vi "Main v1.95.vi"() -> ()   [LabVIEW 2017]
doc: "v0.85:\n- Counts for rejects and total\n\nv0.5:\n\n- Added Reject to Manual Mode\n- Send reject pallet cluster during manual mode\n- Run continuous manual happens only when no error has occured"
uses:
  Controls/Main Tabs v0.1.ctl
  Controls/Auto.ctl
  RT/Controls/Auto Delays.ctl
  RT/Controls/Auto Times.ctl
  support/Controls/General Para.ctl
  Controls/UI Data.ctl
  Controls/AVL Auto Time.ctl
  support/Controls/Auto Stats.ctl
  Controls/Logging FGV.ctl
  support/Message Queue/Enqueue Message (Single).vi
  GV/Maintenance GV.vi
  <vilib>/Utility/error.llb/Error Cluster From Error Code.vi
  <vilib>/ErrorRing/Error Ring.xnode
  support/Message Queue/Message Queue.lvlib
  support/User Event - Stop/User Event - Stop.lvlib
panel:
  out "Rejects 2":u32 caption="Rejects"
  in  "Reset MCount":bool
  out "Output Count":u32 caption="Output\nCount"
  out "OEE":dbl format="%#.1f"
  out "QUA":dbl=100.0 min=0.0 max=100.0 step=0.1
  in  "Ideal Time":dbl=2.0 min=0.0 max=100.0 step=0.1
  in  "AVL":dbl=100.0 min=0.0 max=100.0 step=0.1
  out "PRF":dbl=100.0 min=0.0 max=100.0 step=0.1
  out "path":path
  out "Shutdown?":bool
  in  "Reject Pallets":T1
  out "Date-Time":string caption="Dip-Tube Assembly Automation (HMI) v1.95"
  out "Main Tab":T2
  in  "All IOs":bool
  in  "Autocycle":T3
  in  "Manual":bool
  in  "Parameters":bool
  in  "Maintenance":bool
  in  "General Para":T4={"Max. Cons."=5.0, "Offset 1"=0.0, "Offset 2"=0.0, "Offset 3"=0.0, "Offset 4"=0.0, "OutputPause"=0.0, "RejectPause"=0.0, "IndexTimeout"=0.0} caption="General" {"Offset 4" format="%.2f"; "Offset 3" format="%.2f"; "Offset 2" format="%.2f"; "Offset 1" format="%.2f"}
  in  "BF Para":cluster{"Delay 1":u32, "Delay 2":u32}={"Delay 1"=1000, "Delay 2"=1000}
  in  "Reject Para":cluster{"Delay":u32}={"Delay"=400}
  in  "PF Para":cluster{"Delay 1":u32, "Delay 2":u32}={"Delay 1"=1000, "Delay 2"=1000}
  in  "Tube Feeder Para":T5={"Delay"=400, "Delay 2"=250, "Max Attempts"=250, "Timeout"=8000} caption="TF Para"
  in  "Agitator Para":cluster{"Delay 1":u32, "Delay 2":u32}={"Delay 1"=400, "Delay 2"=250}
  in  "Insertion Para":cluster{"Delay 1":u32, "Delay 2":u32}={"Delay 1"=1000, "Delay 2"=1000}
  in  "Save Para":bool
  in  "Home Para":bool
  in  "Cutting Para":T6={"Delay"=400, "Delay 2"=250, "Delay 3"=250}
  in  "Meas. Para":T7={"Delay"=500.0, "Mean Length"=188.9, "Tolerance"=1.0}
  in  "Enable BF?":bool
  in  "Enable Agitate?":bool
  in  "Enable Reject?":bool
  in  "Toggle Motor":bool
  in  "Continuous?":bool
  in  "Enable Measure?":bool
  in  "Enable Index?":bool
  in  "Enable PF?":bool
  in  "Manual Para":T8={"Agitator Delays"=[400, 250], "TF Delays"=[700, 800, 2], "Insertion Delays"=[100, 500], "Cutting Delays"=[300, 300, 100], "PF Delays"=[250, 30000], "Measur. Delays"=[500.0, 188.9, 1.0], "Reject Delays"=[500], "BF Delays"=[1000, 1000]}
  in  "Enable Cutting?":bool
  in  "Enable Insertion?":bool
  in  "Run Manual":bool
  in  "Enable TF?":bool
  in  "Home Manual":bool
  out "Status 2":T10
  out "Measurements":T11 {"Height 1" format="%#.2f"; "Height 2" format="%#.2f"; "Height 3" format="%#.2f"; "Height 4" format="%#.2f"}
  in  "ResetRejectCount":bool
  in  "ResetGoodCount":bool
  out "RejectPause":u32 caption="Reject Parts"
  out "GoodPause":u32 caption="Good Parts"
  in  "End Cycle":bool
  out "Statuses":string[][](table)
  in  "All IO":bool
  in  "Stats":bool
  in  "Home AC":bool
  out "Status":string
  out "Good":u32 format="%06.0f"
  out "Cycle Time":dbl format="%0.2f"
  out "Rejects":u32 format="%05.0f"
  in  "View Log":bool
  out "Total Count 2":u32 caption="Total Count"
  out "Avg. Time":dbl caption="Avg. Cycle Time (s)" format="%#.3f"
  out "Output Chart":cluster{"Good Parts":u32, "Reject Parts":u32}(graph)
  out "Reject Count":u32
  out "Good Count":u32
  out "Total Time":dbl caption="Effective Cycle Time (s)" format="%#.3f"
  out "Time Chart":T12(graph)
  out "OEE Chart":T13(graph)
  out "Timestamp":string caption="Date & Timestamp"
  out "Latest Measure.":T14 caption="Latest Measurements" {"Length 1 (mm)" format="%#.2f"}
  out "Auto Times":T9
  in  "Back Stats":bool
  out "OEE 2":T13 caption="Latest Measurements" {"AVL" format="%#.1f"; "PRF" format="%#.1f"; "QUA" format="%#.1f"; "OEE" format="%#.1f"}
  out "Measurement Chart":T15(graph)
  in  "Home IOs":bool
  in  "Back IO":bool
  out "IAS 4":dbl format="%#.3f"
  out "IAS 3":dbl format="%#.3f"
  out "IAS 2":dbl format="%#.3f"
  out "IAS 1":dbl format="%#.3f"
  out "DI 1":T16
  out "DI 2":T17
  out "DO 1":T18
  in  "Exit":bool
  in  "Shutdown":bool
  # "HARMONY VISION DIP-TUBE ASSEMBLY AUTOMATION"
  # "Info"
  # "Delays: Time to wait (in milliseconds) after each action pertaining to each spcific station. Generally this timer starts after the required sensor that is expected either goes OFF or goes ON depending on the action. Some stations have multiple delays which are denoted by numbers relative to the sequence of action before the delay.\n\nTimeout: Maximum time allowed (in milliseconds) for a station to complete its actions.\n\nMax Attempts: Maximum number of attempts at retrying gate open/close.\n\nMean Length: Mean length of parts in the current model (in mm)\n\nTolerance: Acceptable deviation from mean length (in mm)\n\nMax Cons.: Maximum number of consecutive tubes missing on a particular pallet (as detected on measurement station) that will trigger an error and cycle stop.\n\nOffset: Offset factor (in mm) added to the measurement result of each probe.\n\nOutputPause & RejectPause: Countdown of number of parts before triggering an Auto-Pause."
  # "Auto-Pause after"
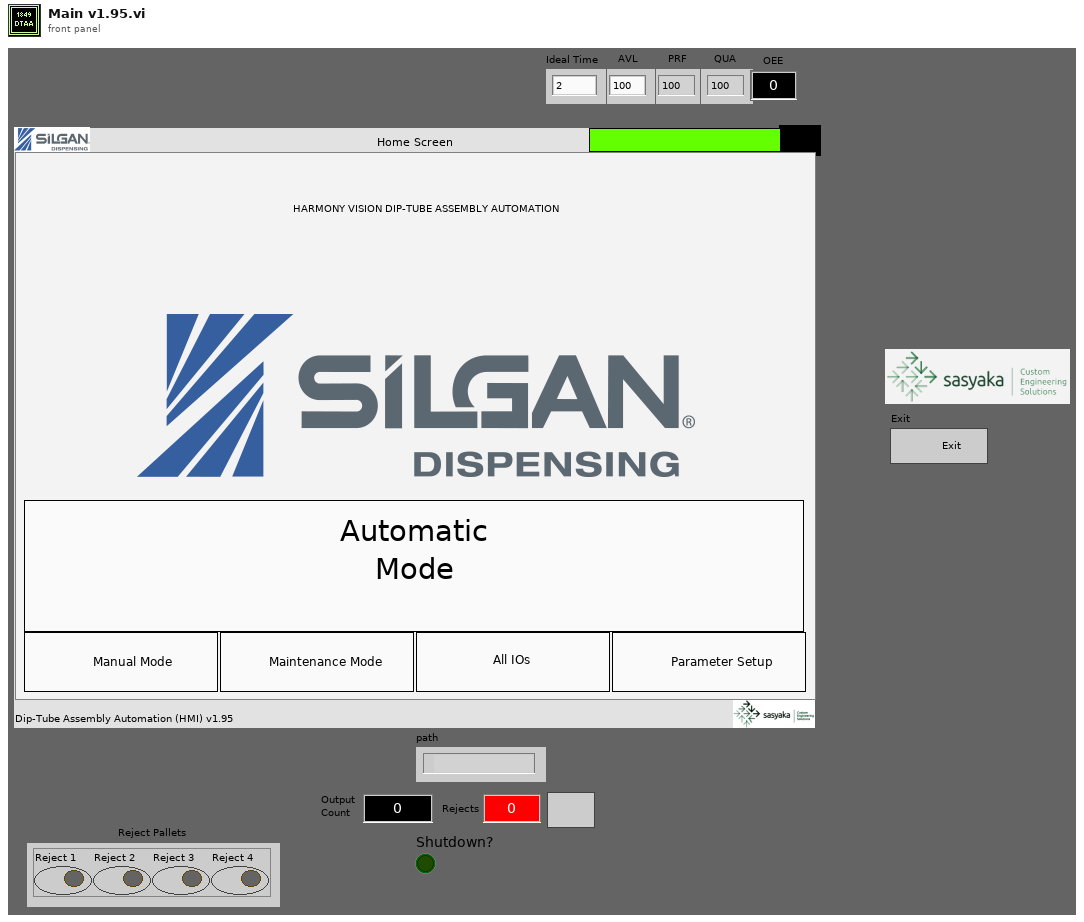
[diagram p1: front panel]
types:
  T1 = cluster{"Reject 1":bool, "Reject 2":bool, "Reject 3":bool, "Reject 4":bool}
  T2 = typedef "Main Tabs v0.1.ctl" = enum32{"Home Screen", "Parameter Setup", "Manual Mode", "Autocycle", "Autocycle Statistics", "Autocycle IOs"}
  T3 = typedef "Auto.ctl" = bool
  T4 = typedef "General Para.ctl" = cluster{"Max. Cons.":dbl, "Offset 1":dbl, "Offset 2":dbl, "Offset 3":dbl, "Offset 4":dbl, "OutputPause":dbl, "RejectPause":dbl, "IndexTimeout":dbl}
  T5 = cluster{"Delay":u32, "Delay 2":u32, "Max Attempts":u32, "Timeout":u32}
  T6 = cluster{"Delay":u32, "Delay 2":u32, "Delay 3":u32}
  T7 = cluster{"Delay":dbl, "Mean Length":dbl, "Tolerance":dbl}
  T8 = typedef "Auto Delays.ctl" = cluster{"Agitator Delays":u32[], "TF Delays":u32[], "Insertion Delays":u32[], "Cutting Delays":u32[], "PF Delays":u32[], "Measur. Delays":dbl[], "Reject Delays":u32[], "BF Delays":u32[]}
  T9 = typedef "Auto Times.ctl" = cluster{"Index Time":u32, "TF Time":u32, "Insertion Time":u32, "Cutting Time":u32, "PF Time":u32, "Meas. Time":u32, "Reject Time":u32}
  T10 = cluster{"Auto Times":T9, "error out":errorcluster}
  T11 = cluster{"Height 1":dbl, "Height 2":dbl, "Height 3":dbl, "Height 4":dbl}
  T12 = cluster{"Index":dbl, "TF":dbl, "Insert":dbl, "Cutting":dbl, "PF":dbl, "Measure.":dbl, "Reject":dbl, "Avg. Cycle Time":dbl}
  T13 = cluster{"AVL":dbl, "PRF":dbl, "QUA":dbl, "OEE":dbl}
  T14 = cluster{"Length 1 (mm)":dbl, "Pallet 2 (mm)":dbl, "Pallet 3 (mm)":dbl, "Pallet 4 (mm)":dbl}
  T15 = cluster{"1":dbl, "2":dbl, "3":dbl, "4":dbl, "4":dbl, "4":dbl}
  T16 = cluster{"Machine_ON":bool, "E_stop ":bool, "SW_Pressure":bool, "SW_Start ":bool, "SW_Reset":bool, "SW_Stop":bool, "SW_Door":bool, "RS_Index_Rotary_CW":bool, "RS_Index_Rotary_CCW":bool, "RS_Index_Stopper _Rear":bool, "RS_Index_Output_Separator_Rear":bool, "PES_Index_Pallet_Sensor":bool, "PES_Index_Output_Part Sensor":bool, "ICS_BF_Low_Level_1":bool, "ICS_BF_Low_Level_2":bool, "ICS_BF_Pump_CNVR_Full_1":bool, "ICS_BF_Pump_CNVR_Full_2":bool, "ICS_BF_Pump_CNVR_Full_3":bool, "ICS_BF_Pump_CNVR_Full_4":bool, "PES_PC_Pump Presence_1":bool, "PES_PC_Pump Presence_2":bool, "PES_PC_Pump Presence_3":bool, "PES_PC_Pump Presence_4":bool, "RS_PC_Gating_Front":bool, "PES_Pump_Interference":bool, "PES_TF_Low_Level":bool, "PES_Tube Presence_1":bool, "PES_Tube Presence_2":bool, "PES_Tube Presence_3":bool, "PES_Tube Presence_4":bool, "DI1.30":bool, "DI1.31":bool}
  T17 = cluster{"RS_Agitatator_1_Rear ":bool, "RS_Agitatator_2_Rear ":bool, "RS_TF_Gating CYL_Rear":bool, "RS_Insertion_1_Rear":bool, "RS_Insertion_1_Front":bool, "RS_Insertion _2_Rear":bool, "RS_Insertion _2_Front":bool, "RS_Insertion _3_Rear":bool, "RS_Insertion _3_Front":bool, "RS_Insertion _4_Rear":bool, "RS_Insertion _4_Front":bool, "RS_Insertion_Clamp_Rear":bool, "RS_Cutting_Rear":bool, "RS_Cutting_Clamp _Rear":bool, "RS_Measurement_1_Rear":bool, "RS_Measurement_2_Rear":bool, "RS_Measurement_3_Rear":bool, "RS_Measurement_4_Rear":bool, "DI2.18":bool, "RS_Rejection_1_Rear":bool, "RS_Rejection_2_Rear":bool, "RS_Rejection_3_Rear":bool, "RS_Rejection_4_Rear":bool, "DI2.23":bool, "DI2.24":bool, "DI2.25":bool, "DI2.26":bool, "DI2.27":bool, "DI2.28":bool, "DI2.29":bool, "DI2.30":bool, "DI2.31":bool}
  T18 = cluster{"TL_Red":bool, "TL_Orange":bool, "TL_Green":bool, "TL_Buzzer":bool, "SOL_Index_Rotary_CW":bool, "SOL_Index_Rotary_CCW":bool, "SOL_Index_Stopper_Rear":bool, "SOL_OutputSeparator_Rear":bool, "Bowl  Feeder_ ON 1":bool, "Pump_CNVR_Motor _ON":bool, "SOL_PC_Gating_CYL_Rear":bool, "SOL_Tube_Feed_Agitatator":bool, "SOL_Tube_Feed_Gating_CYL":bool, "SOL_Insertion _CYL":bool, "SOL_Insertion_Clamp_CYL":bool, "SOL_Cutting_CYL":bool, "SOL_Cutting_Clamp_CYL":bool, "SOL_Insertion_Air_Nozzle":bool, "SOL_Measurement_CYL":bool, "DO1.19":bool, "SOL_Rejection CYL_1":bool, "SOL_Rejection CYL_2":bool, "SOL_Rejection CYL_3":bool, "SOL_Rejection CYL_4":bool, "Bowl  Feeder_ ON 2":bool, "SOL_BF_BlowerON":bool, "SOL_BF1_Track1":bool, "SOL_BF1_Track2":bool, "SOL_BF2_Track1":bool, "SOL_BF2_Track2":bool, "DO1.30":bool, "DO1.31":bool}
  T19 = typedef "UI Data.ctl" = cluster{"Main Tab":refnum<vi>}
  T20 = typedef "Message Queue.lvlib/All Message Queues.ctl" = cluster{"UI":refnum<queue>}
  T21 = enum8{"Enabled", "Disabled", "Disabled and Grayed Out"}
  T22 = typedef "AVL Auto Time.ctl" = enum16{"Start Session", "Exited Auto", "Resumed Auto", "Read Time", "Reload Values"}
  T23 = cluster{"Array":string[][], "Machine Status":string}
  T24 = typedef "Logging FGV.ctl" = enum16{"Start Shift", "Reload Values", "Log Index", "Read Shift", "Close Shift", "Save Values"}
  T25 = typedef "Auto Stats.ctl" = cluster{"Time-Stamp":timestamp, "Auto Times":T9, "Measurements":cluster{"1":dbl, "2":dbl, "3":dbl, "4":dbl}, "Outputs":cluster{"Good Parts":u32, "Reject Parts":u32}, "Cycle Time":dbl, "Remarks":string}
  T26 = cluster{"Auto Times":T9, "Results":cluster{"Measurements":cluster{"1":dbl, "2":dbl, "3":dbl, "4":dbl}, "Reject Pallets":cluster{"Reject 1":bool, "Reject 2":bool, "Reject 3":bool, "Reject 4":bool}}, "OutputCount":u32, "error out":errorcluster}
  T27 = enum8{"Information", "Error", "Successful", "Tips"}
  T28 = cluster{"Agitator Delays[0]":u32, "Agitator Delays[1]":u32}
  T29 = cluster{"TF Delays[0]":u32, "TF Delays[1]":u32, "TF Delays[2]":u32, "TF Delays[3]":u32}
  T30 = cluster{"Insertion Delays[0]":u32, "Insertion Delays[1]":u32}
  T31 = cluster{"Cutting Delays[0]":u32, "Cutting Delays[1]":u32, "Cutting Delays[2]":u32}
  T32 = cluster{"Measur. Delays[0]":dbl, "Measur. Delays[1]":dbl, "Measur. Delays[2]":dbl}
  T33 = typedef "All Inputs.ctl" = cluster{"DI 1":cluster{"Machine_ON":bool, "E_stop ":bool, "SW_Pressure":bool, "SW_Start ":bool, "SW_Reset":bool, "SW_Stop":bool, "SW_Door":bool, "RS_Index_Rotary_CW":bool, "RS_Index_Rotary_CCW":bool, "RS_Index_Stopper _Rear":bool, "RS_Cutting_DNClamp _Rear":bool, "PES_Index_Pallet_Sensor":bool, "PES_Index_Output_Part Sensor":bool, "ICS_BF_Low_Level_1":bool, "ICS_BF_Low_Level_2":bool, "ICS_BF_Pump_CNVR_Full_1":bool, "ICS_BF_Pump_CNVR_Full_2":bool, "ICS_BF_Pump_CNVR_Full_3":bool, "ICS_BF_Pump_CNVR_Full_4":bool, "PES_PC_Pump Presence_1":bool, "PES_PC_Pump Presence_2":bool, "PES_PC_Pump Presence_3":bool, "PES_PC_Pump Presence_4":bool, "RS_PC_Gating_Front":bool, "PES_Pump_Interference":bool, "PES_TF_Low_Level":bool, "PES_Tube Presence_1":bool, "PES_Tube Presence_2":bool, "PES_Tube Presence_3":bool, "PES_Tube Presence_4":bool, "DI1.30":bool, "DI1.31":bool}, "DI 2":cluster{"RS_Agitatator_1_Rear ":bool, "RS_Agitatator_2_Rear ":bool, "RS_TF_Gating CYL_Rear":bool, "RS_Insertion_1_Rear":bool, "RS_Insertion_1_Front":bool, "RS_Insertion _2_Rear":bool, "RS_Insertion _2_Front":bool, "RS_Insertion _3_Rear":bool, "RS_Insertion _3_Front":bool, "RS_Insertion _4_Rear":bool, "RS_Insertion _4_Front":bool, "RS_Insertion_Clamp_Rear":bool, "RS_Cutting_Rear":bool, "RS_Cutting_UPClamp _Rear":bool, "RS_Measurement_1_Rear":bool, "RS_Measurement_2_Rear":bool, "RS_Measurement_3_Rear":bool, "RS_Measurement_4_Rear":bool, "RS_Measure_Clamp_Rear":bool, "RS_Rejection_1_Rear":bool, "RS_Rejection_2_Rear":bool, "RS_Rejection_3_Rear":bool, "RS_Rejection_4_Rear":bool, "DI2.23":bool, "DI2.24":bool, "DI2.25":bool, "DI2.26":bool, "DI2.27":bool, "DI2.28":bool, "DI2.29":bool, "DI2.30":bool, "DI2.31":bool}, "IAS 1":dbl, "IAS 2":dbl, "IAS 3":dbl, "IAS 4":dbl, "DO 1":cluster{"TL_Red":bool, "TL_Orange":bool, "TL_Green":bool, "TL_Buzzer":bool, "SOL_Index_Rotary_CW":bool, "SOL_Index_CNVR_Rotary_CCW":bool, "SOL_Index_CNVR_Stopper_Rear":bool, "SOL_Index_CNVR_Output _Separator _Rear":bool, "Bowl  Feeder_ ON 1":bool, "Pump_CNVR_Motor _ON":bool, "SOL_PC_Gating_CYL_Rear":bool, "SOL_Tube_Feed_Agitatator":bool, "SOL_Tube_Feed_Gating_CYL":bool, "SOL_Insertion _CYL":bool, "SOL_Insertion_Clamp_CYL":bool, "SOL_Cutting_CYL":bool, "SOL_Cutting_Clamp_CYL":bool, "SOL_Insertion_Air_Nozzle":bool, "SOL_Measurement_CYL":bool, "DO1.19":bool, "SOL_Rejection CYL_1":bool, "SOL_Rejection CYL_2":bool, "SOL_Rejection CYL_3":bool, "SOL_Rejection CYL_4":bool, "Bowl  Feeder_ ON 2":bool, "SOL_BF_BlowerON":bool, "SOL_BF1_Track1":bool, "SOL_BF1_Track2":bool, "SOL_BF2_Track1":bool, "SOL_BF2_Track2":bool, "DO1.30":bool, "DO1.31":bool}}
  T34 = cluster{"Machine_ON":bool, "E_stop ":bool, "SW_Pressure":bool, "SW_Start ":bool, "SW_Reset":bool, "SW_Stop":bool, "SW_Door":bool, "RS_Index_Rotary_CW":bool, "RS_Index_Rotary_CCW":bool, "RS_Index_Stopper _Rear":bool, "RS_Cutting_DNClamp _Rear":bool, "PES_Index_Pallet_Sensor":bool, "PES_Index_Output_Part Sensor":bool, "ICS_BF_Low_Level_1":bool, "ICS_BF_Low_Level_2":bool, "ICS_BF_Pump_CNVR_Full_1":bool, "ICS_BF_Pump_CNVR_Full_2":bool, "ICS_BF_Pump_CNVR_Full_3":bool, "ICS_BF_Pump_CNVR_Full_4":bool, "PES_PC_Pump Presence_1":bool, "PES_PC_Pump Presence_2":bool, "PES_PC_Pump Presence_3":bool, "PES_PC_Pump Presence_4":bool, "RS_PC_Gating_Front":bool, "PES_Pump_Interference":bool, "PES_TF_Low_Level":bool, "PES_Tube Presence_1":bool, "PES_Tube Presence_2":bool, "PES_Tube Presence_3":bool, "PES_Tube Presence_4":bool, "DI1.30":bool, "DI1.31":bool}
  T35 = cluster{"RS_Agitatator_1_Rear ":bool, "RS_Agitatator_2_Rear ":bool, "RS_TF_Gating CYL_Rear":bool, "RS_Insertion_1_Rear":bool, "RS_Insertion_1_Front":bool, "RS_Insertion _2_Rear":bool, "RS_Insertion _2_Front":bool, "RS_Insertion _3_Rear":bool, "RS_Insertion _3_Front":bool, "RS_Insertion _4_Rear":bool, "RS_Insertion _4_Front":bool, "RS_Insertion_Clamp_Rear":bool, "RS_Cutting_Rear":bool, "RS_Cutting_UPClamp _Rear":bool, "RS_Measurement_1_Rear":bool, "RS_Measurement_2_Rear":bool, "RS_Measurement_3_Rear":bool, "RS_Measurement_4_Rear":bool, "RS_Measure_Clamp_Rear":bool, "RS_Rejection_1_Rear":bool, "RS_Rejection_2_Rear":bool, "RS_Rejection_3_Rear":bool, "RS_Rejection_4_Rear":bool, "DI2.23":bool, "DI2.24":bool, "DI2.25":bool, "DI2.26":bool, "DI2.27":bool, "DI2.28":bool, "DI2.29":bool, "DI2.30":bool, "DI2.31":bool}
  T36 = cluster{"TL_Red":bool, "TL_Orange":bool, "TL_Green":bool, "TL_Buzzer":bool, "SOL_Index_Rotary_CW":bool, "SOL_Index_CNVR_Rotary_CCW":bool, "SOL_Index_CNVR_Stopper_Rear":bool, "SOL_Index_CNVR_Output _Separator _Rear":bool, "Bowl  Feeder_ ON 1":bool, "Pump_CNVR_Motor _ON":bool, "SOL_PC_Gating_CYL_Rear":bool, "SOL_Tube_Feed_Agitatator":bool, "SOL_Tube_Feed_Gating_CYL":bool, "SOL_Insertion _CYL":bool, "SOL_Insertion_Clamp_CYL":bool, "SOL_Cutting_CYL":bool, "SOL_Cutting_Clamp_CYL":bool, "SOL_Insertion_Air_Nozzle":bool, "SOL_Measurement_CYL":bool, "DO1.19":bool, "SOL_Rejection CYL_1":bool, "SOL_Rejection CYL_2":bool, "SOL_Rejection CYL_3":bool, "SOL_Rejection CYL_4":bool, "Bowl  Feeder_ ON 2":bool, "SOL_BF_BlowerON":bool, "SOL_BF1_Track1":bool, "SOL_BF1_Track2":bool, "SOL_BF2_Track1":bool, "SOL_BF2_Track2":bool, "DO1.30":bool, "DO1.31":bool}
  T37 = cluster{"Index":dbl, "TF":dbl, "Insert":dbl, "Cutting":dbl, "PF":dbl, "Measure.":dbl, "Reject":dbl}
  T38 = cluster{"1":dbl, "2":dbl, "3":dbl, "4":dbl, dbl, dbl}
  T39 = cluster{"Manual Para":T8, "Reject Pallets":cluster{"Reject 1":bool, "Reject 2":bool, "Reject 3":bool, "Reject 4":bool}}
  T40 = cluster{"Measurements":cluster{"1":dbl, "2":dbl, "3":dbl, "4":dbl}, "Reject Pallets":cluster{"Reject 1":bool, "Reject 2":bool, "Reject 3":bool, "Reject 4":bool}}
  T41 = cluster{"Reject Pallets":cluster{"Reject 1":bool, "Reject 2":bool, "Reject 3":bool, "Reject 4":bool}, "Measurements":cluster{"1":dbl, "2":dbl, "3":dbl, "4":dbl}}
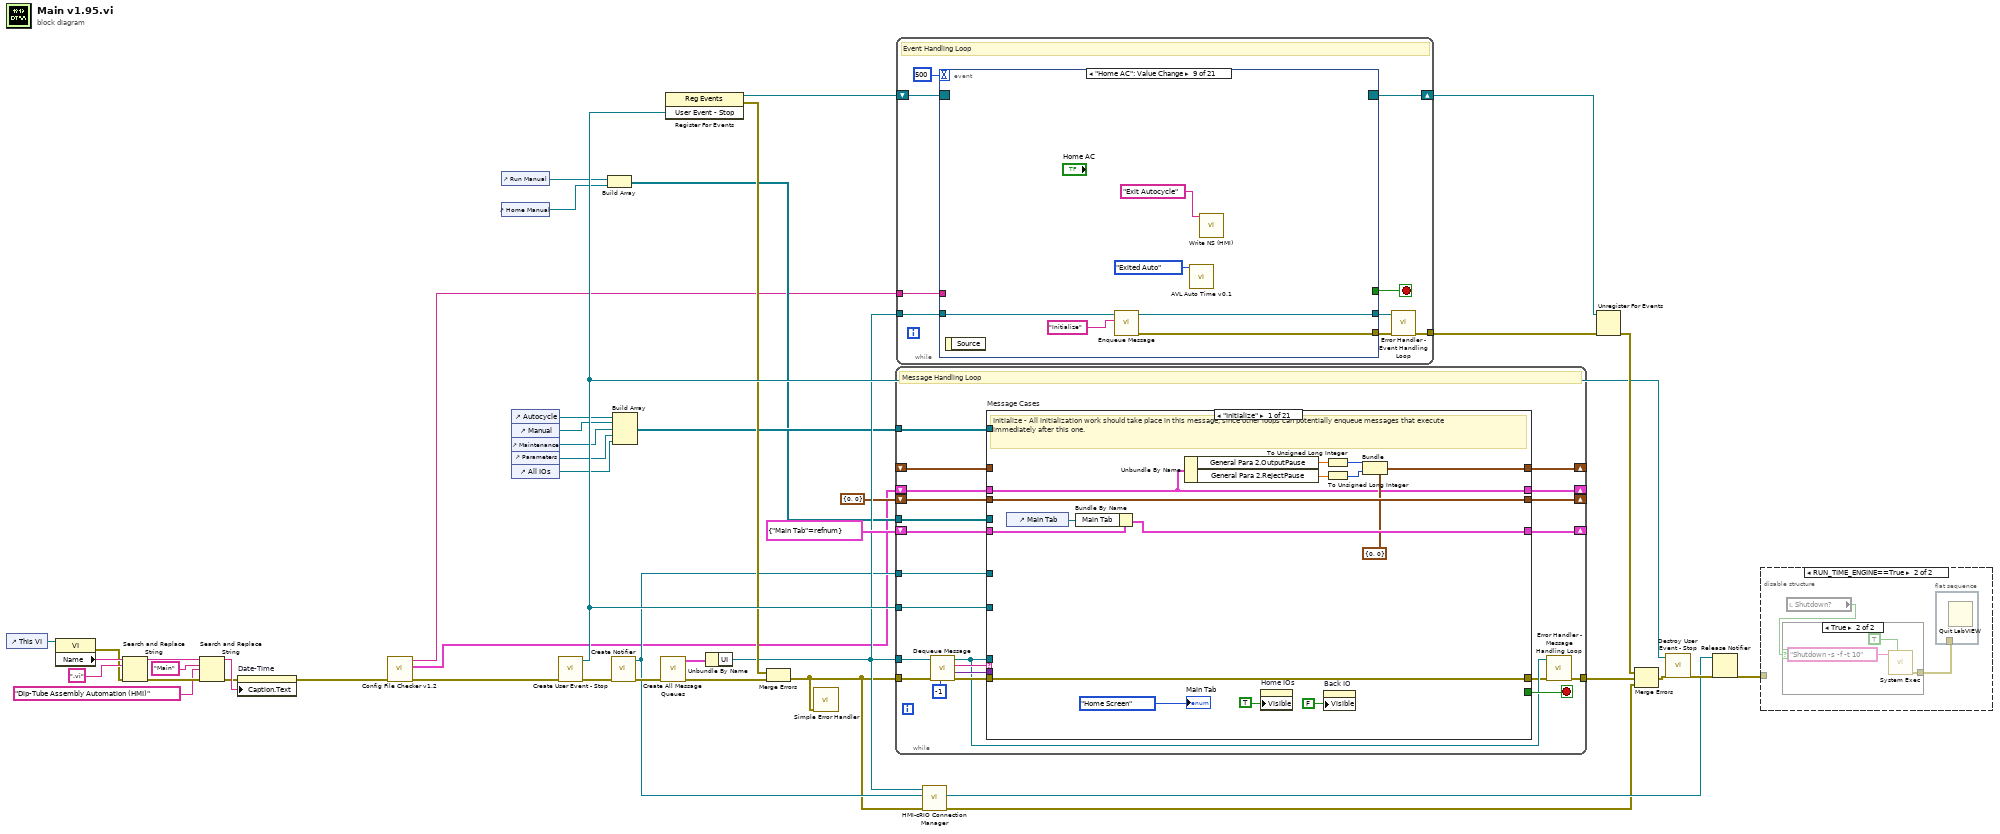
[diagram p0: block diagram]
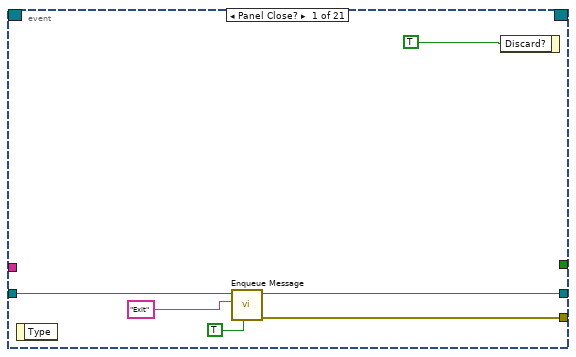
[diagram p2: hidden frame]
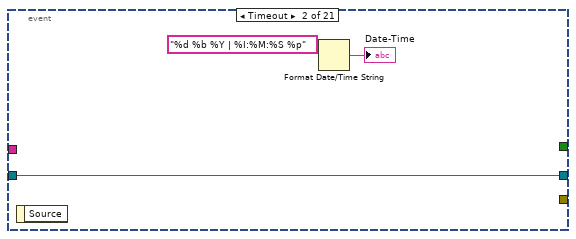
[diagram p3: hidden frame]
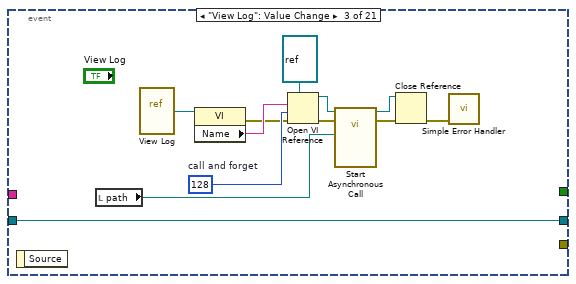
[diagram p4: hidden frame]
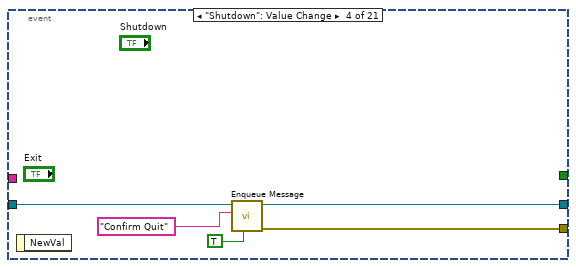
[diagram p5: hidden frame]
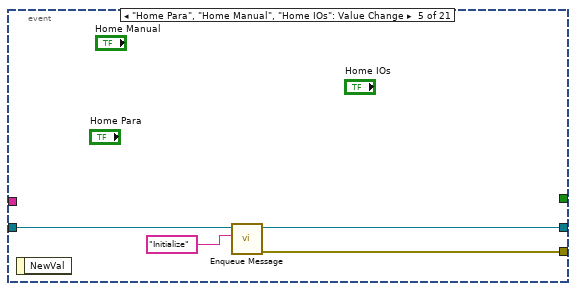
[diagram p6: hidden frame]
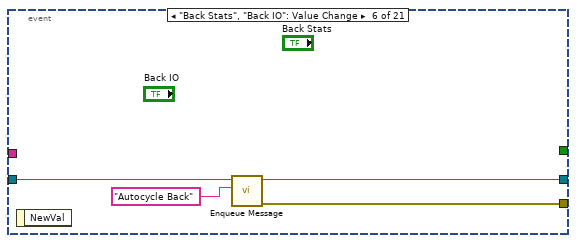
[diagram p7: hidden frame]
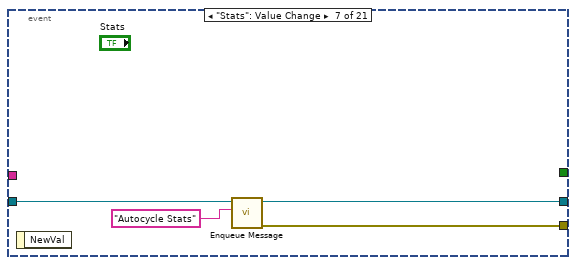
[diagram p8: hidden frame]
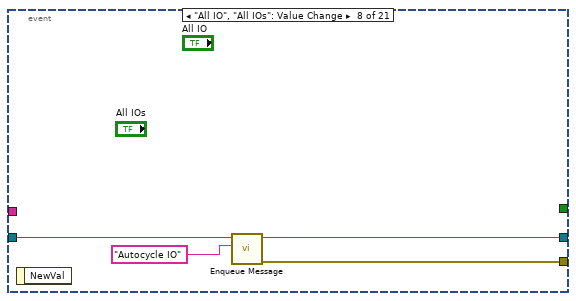
[diagram p9: hidden frame]
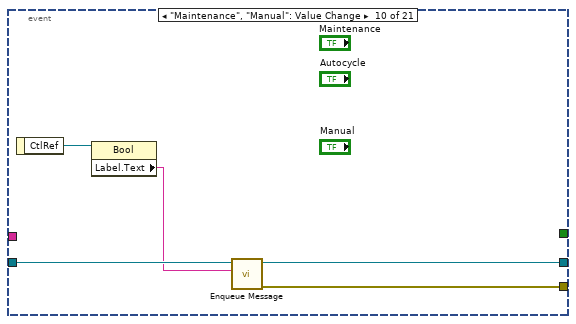
[diagram p10: hidden frame]
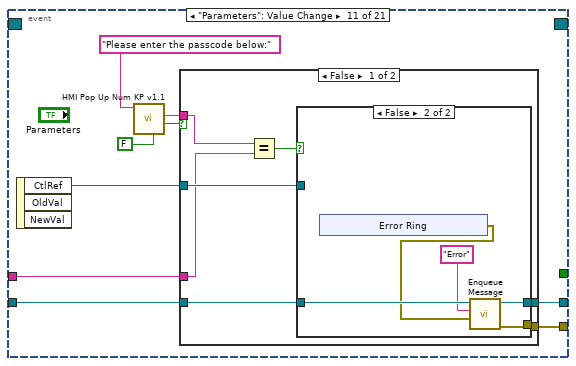
[diagram p11: hidden frame]
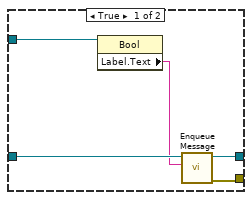
[diagram p12: hidden frame]
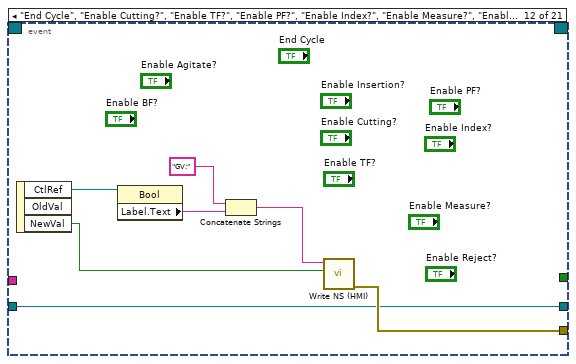
[diagram p14: hidden frame]
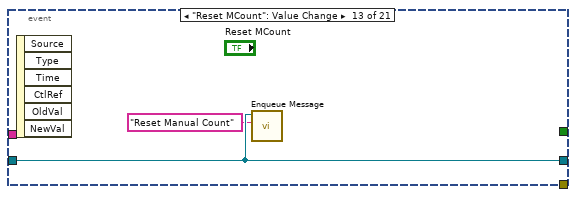
[diagram p15: hidden frame]
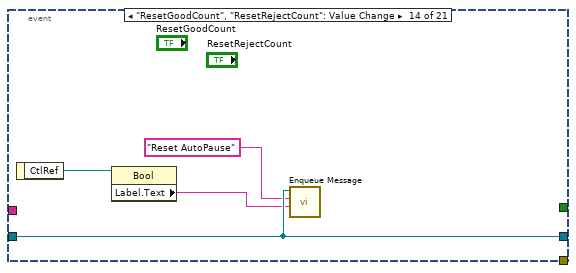
[diagram p16: hidden frame]
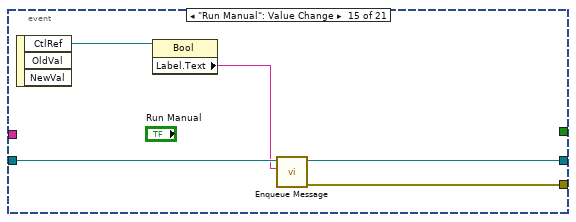
[diagram p17: hidden frame]
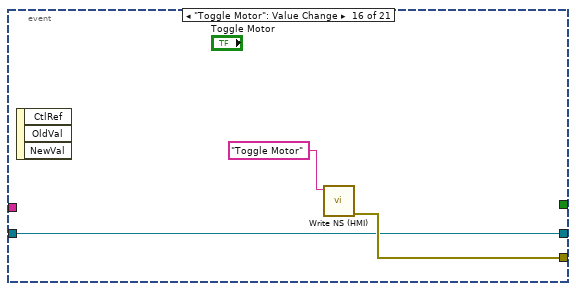
[diagram p18: hidden frame]
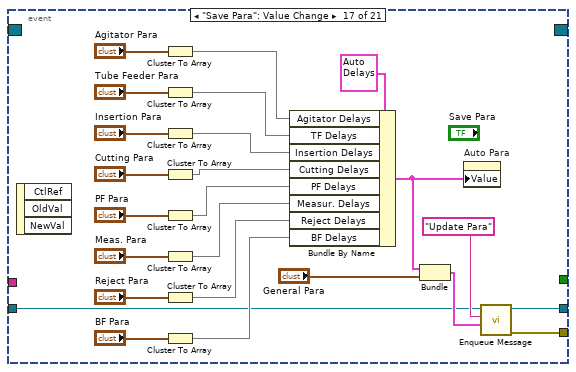
[diagram p19: hidden frame]
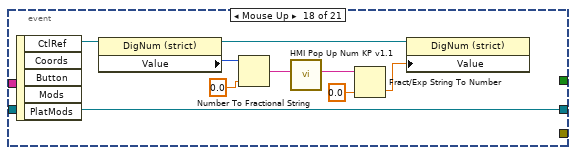
[diagram p20: hidden frame]
diagram:
  n1 = control-ref of="This VI"() -> (w15:refnum<vi>)
  n2 = property class="VI"(reference=w15) -> (error out=w14:errorcluster, "Name"=w21:string)  [unwired: 1 in, 1 out]
  n3 = Search and Replace String(input string=w21, search string=".vi", error in=w14) -> (result string=w19:string, error out=w18:errorcluster)  [unwired: 5 in, 2 out]
  n4 = Search and Replace String(input string=w19, search string="Main", replace string="Dip-Tube Assembly Automation (HMI)" ("replace string (\"\")"), error in=w18) -> (result string=w13:string, error out=w12:errorcluster)  [unwired: 4 in, 2 out]
  n5 = property on="Date-Time" class="Str"(error in=w12, "Caption.Text"=w13) -> (error out=w5:errorcluster)  [unwired: 1 in, 1 out]
  n6 = call "Config File Checker v1.2.vi"("Error In"=w5) -> ("error out"=w4:errorcluster, "All Para"=w1:cluster{"Auto Para":T8, "General Para 2":T4}, "password"=w3:string)  [unwired: 7 in, 1 out]
  n7 = control-ref of="Run Manual"() -> (w11:refnum<vi>)
  n8 = control-ref of="Home Manual"() -> (w10:refnum<vi>)
  n9 = control-ref of="Autocycle"() -> (w26:refnum<vi>)
  n10 = control-ref of="Manual"() -> (w25:refnum<vi>)
  n11 = control-ref of="Maintenance"() -> (w24:refnum<vi>)
  n12 = control-ref of="Parameters"() -> (w23:refnum<vi>)
  n13 = control-ref of="All IOs"() -> (w6:refnum<vi>)
  n14 = call "Create User Event - Stop.vi"("error in (no error)"=w4) -> ("error out"=w32:errorcluster, "User Event - Stop"=w35:refnum<user-event>)  [unwired: 9 in]
  n15 = Build Array(w11, w10) -> (w9:refnum<vi>[])
  n16 = call "Create Notifier.vi"("error in (no error)"=w32) -> ("error out"=w31:errorcluster, "notifier out"=w7:refnum<notifier>)  [unwired: 9 in]
  n17 = Build Array(w26, w25, w24, w23, w6) -> (w22:refnum<vi>[])
  n18 = call "Create All Message Queues.vi"("error in (no error)"=w31) -> ("error out"=w44:errorcluster, "Message Queues out"=w43:T20)  [unwired: 9 in]
  n19 = register-events(w35) -> (reference out=w36:refnum<event-registration>, error out=w34:errorcluster)  [unwired: 2 in]
  n20 = Unbundle By Name(w43) -> ("UI"=w33:refnum<queue>)
  n21 = Merge Errors(w34, w44) -> (w2:errorcluster)
  n22 = call <vilib>:"Simple Error Handler.vi"("error in (no error)"=w2) -> ()  [unwired: 4 in, 5 out]
  n23 = while {
    tunnel: w33 -> [w59]
    shift-right: [w66] -> _
    shift-left: T19 {"Main Tab"=refnum} ("Data Cluster") -> [w49]
    tunnel: w35 -> [w64]
    tunnel: w2 -> [w63]
    tunnel: [w57] -> w42
    tunnel: w7 -> [w54]
    tunnel: w22 -> [w53]
    tunnel: w9 -> [w52]
    shift-right: [w50] -> _
    shift-left: cluster{"OutputCount":u32, "RejectCount":u32} {"OutputCount"=0, "RejectCount"=0} -> [w51]
    shift-right: [w47] -> _
    shift-left: w1 -> [w48]
    shift-right: [w45] -> _
    shift-left: _ -> [w46]
    stop <- w65 stop-if-true
    # "Message Handling Loop"
    n24 = call "Dequeue Message.vi"("timeout"=-1, "error in (no error)"=w63, "Message Queue"=w59) -> ("error out"=w62:errorcluster, "Message Data"=w60:variant, "Message"=w61:string, "dup Message Queue"=w58:refnum<queue>)  [unwired: 5 in]
    n25 = case "Message Cases" shown="\"Initialize\"" w61 {
      selector: w61 -> [_ _ _ _ _ _ _ _ _ _ _ _ _ _ _ _ _ _ _ _ w470]
      tunnel: w58 -> [_ _ _ _ _ _ _ _ _ w225 w235 _ w280 _ w361 _ _ _ w438 w466 _]
      tunnel: w62 -> [w81 w86 w102 w132 w149 w167 w178 w211 w218 w227 w243 w273 w323 w335 w369 w381 w391 w428 w442 w459 _]
      tunnel: [w81 w85 w91 w132 w144 w167 w177 w211 w218 w226 w242 w274 w324 w337 w360 w381 w390 w423 w440 w462 w471] -> w56
      tunnel: w49 -> [w80 w87 w104 w136 w151 w166 w174 w215 w222 w232 w240 w275 w325 w338 w370 w380 w393 w427 w441 w465 w472]
      tunnel: [w79 w87 w104 w136 w151 w166 w174 w215 w222 w232 w240 w275 w325 w338 w370 w380 w393 w427 w441 w465 w472] -> w66
      tunnel: [_ _ _ _ _ _ _ _ _ _ _ _ _ _ _ _ _ _ _ TRUE _] -> w65
      tunnel: w60 -> [_ _ w101 _ w148 _ _ _ _ _ _ w272 w322 _ w368 _ w389 w426 _ w456 _]
      tunnel: w64 -> [_ _ _ _ _ _ _ _ _ _ _ _ _ _ _ _ _ _ _ w461 _]
      tunnel: w54 -> [_ _ _ _ _ _ _ _ _ _ _ _ _ _ _ _ _ _ _ w455 _]
      tunnel: w53 -> [_ _ w97 _ _ _ _ _ _ _ _ _ _ _ _ _ _ _ _ _ _]
      tunnel: w52 -> [_ _ _ _ _ _ _ _ _ _ _ _ _ w332 w366 _ _ _ _ _ _]
      tunnel: w51 -> [w76 w84 w93 w133 w150 w155 w179 w212 w219 w229 w244 w270 w320 w328 w359 _ w392 w422 w437 w452 w469]
      tunnel: [w76 w84 w93 w133 w150 w155 w179 w212 w219 w229 w244 w270 w320 w328 w354 cluster{"OutputCount":u32, "RejectCount":u32} {"OutputCount"=0, "RejectCount"=0} w392 w422 w437 w452 w469] -> w50
      tunnel: w48 -> [w68 w83 w90 w113 _ w154 w173 w210 w217 w224 w234 w259 w289 w327 w342 w377 w385 w405 w430 w451 w468]
      tunnel: [w68 w83 w90 w113 w143 w154 w173 w210 w217 w224 w234 w259 w289 w327 w342 w377 w385 w405 w430 w451 w468] -> w47
      tunnel: w46 -> [_ w82 w88 w112 w137 w152 w170 w209 w216 w223 w233 w258 w281 w326 w341 w376 w386 w404 w429 w450 w467]
      tunnel: [w67 w82 w88 w112 w137 w152 w171 w209 w216 w223 w233 w258 w278 w326 w341 w376 w384 w404 w429 w450 w467] -> w45
      frame "Initialize" {
        # "Initialize - All initialization work should take place in this message, since other loops can potentially enqueue messages that execute immediately after this one."
        n26 = control-ref of="Main Tab"() -> (w78:refnum<vi>)
        n27 = Bundle By Name(cluster=w80, "Main Tab"=w78) -> (w79:T19)
        n28 = Unbundle By Name(w68) -> ("General Para 2.OutputPause"=w71:dbl, "General Para 2.RejectPause"=w70:dbl)
        n29 = property on="Home IOs" class="Bool"("Visible"=TRUE) -> ()  [unwired: 2 in, 2 out]
        n30 = property on="Back IO" class="Bool"("Visible"=FALSE) -> ()  [unwired: 2 in, 2 out]
        n31 = To Unsigned Long Integer(number=w71) -> (unsigned 32bit integer=w72:u32)
        n32 = To Unsigned Long Integer(number=w70) -> (unsigned 32bit integer=w73:u32)
        n33 = Bundle(cluster=cluster{"GoodPause":u32, "RejectPause":u32} {"GoodPause"=0, "RejectPause"=0}, "GoodPause"=w72, "RejectPause"=w73) -> (w67:cluster{"GoodPause":u32, "RejectPause":u32})
        "Main Tab" <- Main_Tabs_v0.1."Home Screen" ("Main Tab")
      }
      frame "Maintenance" {
        # "Maintenance"
        n34 = call "Maintenance v0.3.vi"("Error In"=w86) -> ("Error out"=w85:errorcluster)  [unwired: 10 in]
      }
      frame "Connection" {
        n35 = Variant To Data(error in=w102, type=FALSE, Variant=w101) -> (data=w89:bool, error out=w92:errorcluster)
        n36 = Select(t=u32 6618880 ("Text.Text Colors:BG Color"), s=w89, f=u32 16762112 ("Text.Text Colors:BG Color")) -> (s? t:f=w98:u32)
        n37 = property on="Date-Time" class="Str"("Text.BGColor"=w98) -> ()  [unwired: 2 in, 2 out]
        n38 = Select(t=T21."Enabled" ("Disabled"), s=w89, f=T21."Disabled and Grayed Out") -> (s? t:f=w95:T21)
        n39 = for {
          tunnel: w97 -> [w111] mode=indexing
          tunnel: w95 -> [w110]
          n40 = property class="Bool"(reference=w111, "DisabledEnum"=w110) -> ()  [unwired: 1 in, 2 out]
        }
        n41 = case shown="True" w89 {
          tunnel: w92 -> [w105 w108]
          tunnel: [w105 w107] -> w91
          tunnel: w90 -> [_ w106]
          frame False {
          }
          frame True {
            n42 = call "Write NS (HMI).vi"("error in (no error)"=w108, "Message Data"=w106, "Message"="Save Para") -> ("error out"=w107:errorcluster)  [unwired: 8 in]
          }
        }
      }
      frame "Parameters" {
        # "Parameters"
        n43 = Unbundle(w113) -> ("Auto Para"=w115:T8, "General Para 2"=w114:T4)
        n44 = Unbundle By Name(w136) -> ("Main Tab"=w135:refnum<vi>)
        n45 = property on="General Para" class="Clust (strict)"("Value"=w114) -> ()  [unwired: 2 in, 2 out]
        n46 = Unbundle(w115) -> ("Agitator Delays"=w131:u32[], "TF Delays"=w130:u32[], "Insertion Delays"=w129:u32[], "Cutting Delays"=w128:u32[], "PF Delays"=w127:u32[], "Measur. Delays"=w126:dbl[], "Reject Delays"=w125:u32[], "BF Delays"=w124:u32[])
        n47 = property class="TabCtl"(reference=w135, "Value"=Main_Tabs_v0.1."Parameter Setup" ("Main Tab")) -> ()  [unwired: 1 in, 2 out]
        n48 = Array To Cluster(array=w131) -> (cluster=w123:T28)
        n49 = Array To Cluster(array=w130) -> (cluster=w122:T29)
        n50 = Array To Cluster(array=w129) -> (cluster=w121:T30)
        n51 = Array To Cluster(array=w128) -> (cluster=w120:T31)
        n52 = Array To Cluster(array=w127) -> (cluster=w119:cluster{"PF Delays[0]":u32, "PF Delays[1]":u32})
        n53 = Array To Cluster(array=w126) -> (cluster=w118:T32)
        n54 = Array To Cluster(array=w125) -> (cluster=w117:cluster{"Reject Delays[0]":u32})
        n55 = Array To Cluster(array=w124) -> (cluster=w116:cluster{"BF Delays[0]":u32, "BF Delays[1]":u32})
        n56 = property on="Agitator Para" class="Clust (strict)"("Value"=w123) -> ()  [unwired: 2 in, 2 out]
        n57 = property on="Tube Feeder Para" class="Clust (strict)"("Value"=w122) -> ()  [unwired: 2 in, 2 out]
        n58 = property on="Insertion Para" class="Clust (strict)"("Value"=w121) -> ()  [unwired: 2 in, 2 out]
        n59 = property on="Cutting Para" class="Clust (strict)"("Value"=w120) -> ()  [unwired: 2 in, 2 out]
        n60 = property on="PF Para" class="Clust (strict)"("Value"=w119) -> ()  [unwired: 2 in, 2 out]
        n61 = property on="Meas. Para" class="Clust (strict)"("Value"=w118) -> ()  [unwired: 2 in, 2 out]
        n62 = property on="Reject Para" class="Clust (strict)"("Value"=w117) -> ()  [unwired: 2 in, 2 out]
        n63 = property on="BF Para" class="Clust (strict)"("Value"=w116) -> ()  [unwired: 2 in, 2 out]
      }
      frame "Update Para" {
        # "Parameters"
        n64 = Variant To Data(error in=w149, type=cluster{"Auto Para":T8, "General Para":T4} {"Auto Para"={"Agitator Delays"=[], "TF Delays"=[], "Insertion Delays"=[], "Cutting Delays"=[], "PF Delays"=[], "Measur. Delays"=[], "Reject Delays"=[], "BF Delays"=[]}, "General Para"={"Max. Cons."=0.0, "Offset 1"=0.0, "Offset 2"=0.0, "Offset 3"=0.0, "Offset 4"=0.0, "OutputPause"=0.0, "RejectPause"=0.0, "IndexTimeout"=0.0}} ("cluster"), Variant=w148) -> (data=w143:cluster{"Auto Para":T8, "General Para":T4}, error out=w145:errorcluster)
        n65 = call <vilib>:"Application Directory.vi"() -> ("Application Directory"=w142:path)
        n66 = Build Path(base path=w142, name or relative path="data") -> (appended path=w140:path)
        n67 = Build Path(base path=w140, name or relative path="config.ini") -> (appended path=w139:path)
        n68 = call "Write NS (HMI).vi"("error in (no error)"=w145, "Message Data"=w143, "Message"="Save Para") -> ("error out"=w144:errorcluster)  [unwired: 8 in]
        n69 = call "Write Config v1.1.vi"("All Para"=w143, "file path"=w139) -> ()  [unwired: 8 in, 2 out]
      }
      frame "Manual" {
        # "Parameters"
        n70 = control-ref of="Enable Index?"() -> (w163:refnum<vi>)
        n71 = control-ref of="Enable PF?"() -> (w162:refnum<vi>)
        n72 = control-ref of="Enable Cutting?"() -> (w161:refnum<vi>)
        n73 = control-ref of="Enable Insertion?"() -> (w160:refnum<vi>)
        n74 = control-ref of="Enable TF?"() -> (w159:refnum<vi>)
        n75 = control-ref of="Enable Measure?"() -> (w157:refnum<vi>)
        n76 = Unbundle By Name(w154) -> ("Auto Para"=w153:T8)
        n77 = control-ref of="Enable Reject?"() -> (w156:refnum<vi>)
        n78 = Build Array(w163, w162, w161, w160, w159, w157, w156) -> (w158:refnum<vi>[])
        n79 = property on="Auto Para" class="Clust (strict)"("Value"=w153) -> ()  [unwired: 2 in, 2 out]
        n80 = for {
          tunnel: w158 -> [w169] mode=indexing
          n81 = property class="Bool (strict)"(reference=w169, "Val(Sgnl)"=FALSE ("Value (Signaling)")) -> ()  [unwired: 1 in, 2 out]
        }
        n82 = Unbundle By Name(w166) -> ("Main Tab"=w165:refnum<vi>)
        n83 = property class="TabCtl"(reference=w165, "Value"=Main_Tabs_v0.1."Manual Mode" ("Main Tab")) -> ()  [unwired: 1 in, 2 out]
      }
      frame "Autocycle" {
        # "Parameters"
        n84 = call "Select Model v0.1.vi"() -> ("Cancel out"=w175:bool, "Refresh Indicators?"=w172:bool, "Model out"=w176:string)  [unwired: 9 in]
        n85 = case shown="False" w175 {
          tunnel: w178 -> [w192 w208]
          tunnel: [w199 w208] -> w177
          tunnel: w176 -> [w198 _]
          tunnel: w174 -> [w195 _]
          tunnel: w173 -> [w189 _]
          tunnel: w172 -> [w183 _]
          tunnel: [w182 w207] -> w171
          tunnel: w170 -> [w184 w207]
          frame False {
            n86 = Unbundle By Name(w189) -> ("General Para 2.OutputPause"=w188:dbl, "General Para 2.RejectPause"=w187:dbl)
            n87 = Unbundle By Name(w195) -> ("Main Tab"=w197:refnum<vi>)
            n88 = call "Write NS (HMI).vi"("error in (no error)"=w192, "Message Data"=w189, "Message"="Save Para") -> ("error out"=w191:errorcluster)  [unwired: 8 in]
            n89 = property class="TabCtl"(reference=w197, "Value"=Main_Tabs_v0.1."Autocycle" ("Main Tab")) -> ()  [unwired: 1 in, 2 out]
            n90 = call "Write NS (HMI).vi"("error in (no error)"=w191, "Message Data"=w198, "Message"="Autocycle") -> ("error out"=w199:errorcluster)  [unwired: 8 in]
            n91 = property on="Home IOs" class="Bool"("Visible"=FALSE) -> ()  [unwired: 2 in, 2 out]
            n92 = To Unsigned Long Integer(number=w188) -> (unsigned 32bit integer=w186:u32)
            n93 = To Unsigned Long Integer(number=w187) -> (unsigned 32bit integer=w185:u32)
            n94 = property on="Back IO" class="Bool"("Visible"=TRUE) -> ()  [unwired: 2 in, 2 out]
            n95 = case shown="False" w183 {
              tunnel: [w202 w206] -> w182
              tunnel: w186 -> [_ w203]
              tunnel: w185 -> [_ w204]
              tunnel: w184 -> [w202 w205]
              frame False {
                n96 = call "AVL Auto Time v0.1.vi"("State"=AVL_Auto_Time."Resumed Auto") -> ()  [unwired: 9 in, 2 out]
              }
              frame True {
                n97 = Bundle(cluster=w205, "GoodPause"=w203, "RejectPause"=w204) -> (w206:cluster{"GoodPause":u32, "RejectPause":u32})
              }
            }
            n98 = Unbundle(w182) -> ("GoodPause"=w181:u32, "RejectPause"=w180:u32)
            n99 = local write "RejectPause"(w180) -> ()
            n100 = local write "GoodPause"(w181) -> ()
          }
          frame True {
          }
        }
      }
      frame "Autocycle Back" {
        # "Parameters"
        n101 = Unbundle By Name(w215) -> ("Main Tab"=w214:refnum<vi>)
        n102 = property class="TabCtl"(reference=w214, "Value"=Main_Tabs_v0.1."Autocycle" ("Main Tab")) -> ()  [unwired: 1 in, 2 out]
      }
      frame "Autocycle Stats" {
        # "Parameters"
        n103 = Unbundle By Name(w222) -> ("Main Tab"=w221:refnum<vi>)
        n104 = property class="TabCtl"(reference=w221, "Value"=Main_Tabs_v0.1."Autocycle Statistics" ("Main Tab")) -> ()  [unwired: 1 in, 2 out]
      }
      frame "Autocycle IO" {
        # "Parameters"
        n105 = Unbundle By Name(w232) -> ("Main Tab"=w231:refnum<vi>)
        n106 = property class="TabCtl"(reference=w231, "Value"=Main_Tabs_v0.1."Autocycle IOs" ("Main Tab")) -> ()  [unwired: 1 in, 2 out]
        n107 = call-poly "Enqueue Message.vi"("error in (no error)"=w227, "Message"="Update IO", "Message Queue"=w225) -> ("error out"=w226:errorcluster)  [unwired: 7 in, 1 out]
      }
      frame "Update IO" {
        n108 = Unbundle By Name(w240) -> ("Main Tab"=w241:refnum<vi>)
        n109 = Wait (ms)(milliseconds to wait=u32 200) -> ()  [unwired: 1 out]
        n110 = property class="TabCtl"(reference=w241) -> ("Value"=w239:variant)  [unwired: 1 in, 2 out]
        n111 = Variant To Data(type=Main_Tabs_v0.1."Autocycle IOs" ("Main Tab"), Variant=w239) -> (data=w236:T2)  [unwired: 1 in, 1 out]
        n112 = global read "Maintenance GV.vi" "All IO"() -> (w245:T33)
        n113 = case shown="\"Autocycle IOs\"" w236 {
          tunnel: w243 -> [w253 w256]
          tunnel: [w253 w255] -> w242
          tunnel: w235 -> [_ w254]
          frame Default {
          }
          frame "Autocycle IOs" {
            n114 = call-poly "Enqueue Message.vi"("error in (no error)"=w256, "Message"="Update IO", "Message Queue"=w254) -> ("error out"=w255:errorcluster)  [unwired: 7 in, 1 out]
          }
        }
        n115 = Unbundle(w245) -> ("DI 1"=→"DI 1":T34, "DI 2"=→"DI 2":T35, "IAS 1"=→"IAS 1":dbl, "IAS 2"=→"IAS 2":dbl, "IAS 3"=→"IAS 3":dbl, "IAS 4"=→"IAS 4":dbl, "DO 1"=→"DO 1":T36)
      }
      frame "Update UI" {
        # "Update Display - Convert the message data to a string to display in the Data Display indicator."
        n116 = Variant To Data(error in=w273, type=T23 {"Array"=[], "Machine Status"=""} ("Status Cluster"), Variant=w272) -> (data=w268:T23, error out=w271:errorcluster)
        n117 = Unbundle(w268) -> ("Array"=→"Statuses":string[][], "Machine Status"=w266:string)
        "Status" <- w266
        n118 = Search and Replace String(input string=w266, search string="Autocycle is Running") -> (number of replacements=w264:i32)  [unwired: 6 in, 3 out]
        n119 = Greater Than 0?(x=w264) -> (x > 0?=w262:bool)
        n120 = Select(t=T21."Disabled and Grayed Out" ("Disabled"), s=w262, f=T21."Enabled" ("Disabled")) -> (s? t:f=w261:T21)
        n121 = property on="Home AC" class="Bool"("DisabledEnum"=w261) -> ()  [unwired: 2 in, 2 out]
        n122 = Merge Errors(w271) -> (w274:errorcluster)
      }
      frame "Autocycle Log" {
        # "Update Display - Convert the message data to a string to display in the Data Display indicator."
        n123 = Variant To Data(error in=w323, type=T25 {"Time-Stamp"=timestamp(0 s since 1904-01-01), "Auto Times"={"Index Time"=0, "TF Time"=0, "Insertion Time"=0, "Cutting Time"=0, "PF Time"=0, "Meas. Time"=0, "Reject Time"=0}, "Measurements"={"1"=0.0, "2"=0.0, "3"=0.0, "4"=0.0}, "Outputs"={"Good Parts"=0, "Reject Parts"=0}, "Cycle Time"=0.0, "Remarks"=""} ("Auto Stats"), Variant=w322) -> (data=w279:T25, error out=w321:errorcluster)
        n124 = Unbundle By Name(w279) -> ("Time-Stamp"=w317:timestamp, "Measurements"=w309:cluster{"1":dbl, "2":dbl, "3":dbl, "4":dbl}, "Outputs"=→"Output Chart":cluster{"Good Parts":u32, "Reject Parts":u32}, "Auto Times"=→"Auto Times":T9)
        "Latest Measure." <- w309
        n125 = call "Stats Unbundle v0.2.vi"("State"=Logging_FGV."Log Index", "Auto Stats"=w279) -> ("Cycle Time"=→"Cycle Time" →"Total Time":dbl, "Counters"=w313:cluster{"GoodCount":u32, "RejectCount":u32}, "OEE Cluster"=→"OEE Chart" →"OEE 2":T13, "Avg. Cycle Time"=w291:dbl, "Total Times"=w299:T37, "path"=→"path":path)  [unwired: 3 in, 1 out]
        "Avg. Time" <- w291
        n126 = Format Date/Time String(time format string (%c)="%d-%m-%Y | %H:%M:%S%3u", seconds (now)=w317) -> (date/time string=→"Timestamp":string)  [unwired: 1 in]
        n127 = Unbundle By Name(w289) -> ("Auto Para.Measur. Delays"=w288:dbl[])
        n128 = Unbundle By Name(w313) -> ("GoodCount"=w301:u32, "RejectCount"=w302:u32)
        "Rejects" <- w302
        "Good" <- w301
        "Good Count" <- w301
        "Reject Count" <- w302
        n129 = call "Auto-Pause Check.vi"("Auto Stats"=w279, "Queue"=w280, "Autopause"=w281) -> ("Autopause out"=w278:cluster{"GoodPause":u32, "RejectPause":u32})  [unwired: 8 in]
        n130 = Index Array(array=w288, index #1=1 ("index"), index #2=2 ("index")) -> (element #1=w283:dbl, element #2=w282:dbl)
        n131 = Unbundle(w299) -> ("Index"=w298:dbl, "TF"=w297:dbl, "Insert"=w296:dbl, "Cutting"=w295:dbl, "PF"=w294:dbl, "Measure."=w293:dbl, "Reject"=w292:dbl)
        n132 = Bundle("Index"=w298, "TF"=w297, "Insert"=w296, "Cutting"=w295, "PF"=w294, "Measure."=w293, "Reject"=w292, "Avg. Cycle Time"=w291) -> (→"Time Chart":T12)  [unwired: 1 in]
        n133 = Add(x=w283, y=w282) -> (x+y=w285:dbl)
        n134 = Subtract(x=w283, y=w282) -> (x-y=w284:dbl)
        n135 = Add(x=w301, y=w302) -> (x+y=→"Total Count 2":u32)
        n136 = Unbundle(w309) -> ("1"=w308:dbl, "2"=w307:dbl, "3"=w306:dbl, "4"=w305:dbl)
        n137 = Unbundle(w278) -> ("GoodPause"=→"GoodPause":u32, "RejectPause"=→"RejectPause":u32)
        n138 = Bundle("1"=w308, "2"=w307, "3"=w306, "4"=w305, w285, w284) -> (→"Measurement Chart":T38)  [unwired: 1 in]
        n139 = Merge Errors(w321) -> (w324:errorcluster)
      }
      frame "Run Manual" {
        # "Update Manual mode"
        n140 = Bundle("Manual Para"="Manual Para", "Reject Pallets"="Reject Pallets") -> (w329:T39)  [unwired: 1 in]
        n141 = for {
          tunnel: w332 -> [w340] mode=indexing
          tunnel: T21."Disabled and Grayed Out" ("Disabled") -> [w339]
          n142 = property class="Bool"(reference=w340, "DisabledEnum"=w339) -> ()  [unwired: 1 in, 2 out]
        }
        n143 = call "Write NS (HMI).vi"("error in (no error)"=w335, "Message Data"=w329, "Message"="Manual Run") -> ("error out"=w334:errorcluster)  [unwired: 8 in]
        n144 = Merge Errors(w334) -> (w337:errorcluster)
      }
      frame "Manual Status" {
        n145 = Variant To Data(error in=w369, type=T26 {"Auto Times"={"Index Time"=0, "TF Time"=0, "Insertion Time"=0, "Cutting Time"=0, "PF Time"=0, "Meas. Time"=0, "Reject Time"=0}, "Results"={"Measurements"={"1"=0.0, "2"=0.0, "3"=0.0, "4"=0.0}, "Reject Pallets"={"Reject 1"=FALSE, "Reject 2"=FALSE, "Reject 3"=FALSE, "Reject 4"=FALSE}}, "OutputCount"=0, "error out"={"status"=FALSE, "code"=0, "source"=""}} ("cluster"), Variant=w368) -> (data=w365:T26, error out=w360:errorcluster)
        n146 = Unbundle(w365) -> ("Auto Times"=w364:T9, "Results"=w356:T40, "OutputCount"=w355:u32, "error out"=w358:errorcluster)
        n147 = for {
          tunnel: w366 -> [w375] mode=indexing
          tunnel: T21."Enabled" ("Disabled") -> [w374]
          n148 = property class="Bool"(reference=w375, "DisabledEnum"=w374) -> ()  [unwired: 1 in, 2 out]
        }
        n149 = Unbundle(w356) -> ("Measurements"=w344:cluster{"1":dbl, "2":dbl, "3":dbl, "4":dbl}, "Reject Pallets"=w345:T1)
        "Measurements" <- w344
        n150 = Bundle("Auto Times"=w364, "error out"=w358) -> (→"Status 2":T10)  [unwired: 1 in]
        n151 = Bundle("Reject Pallets"=w345, "Measurements"=w344) -> (w343:T41)  [unwired: 1 in]
        n152 = call "Counts Update (manual).vi"("output cluster"=w343, "Desired Cycle Time (s)"="Ideal Time", "AVL"="AVL", "OutputCount"=w355, "Counts in"=w359) -> ("OEE"=w349:T13, "Counts out"=w354:cluster{"OutputCount":u32, "RejectCount":u32})  [unwired: 5 in]
        n153 = Unbundle(w349) -> ("PRF"=→"PRF":dbl, "QUA"=→"QUA":dbl, "OEE"=→"OEE":dbl)  [unwired: 1 out]
        n154 = Unbundle(w354) -> ("OutputCount"=→"Output Count":u32, "RejectCount"=→"Rejects 2":u32)
        n155 = case shown="True" "Continuous?" {
          tunnel: w361 -> [_ w373]
          tunnel: w358 -> [_ w372]
          frame False {
          }
          frame True {
            # "Run if continuous is TRUE & No Error"
            n156 = call-poly "Enqueue Message.vi"("error in (no error)"=w372, "Message"="Run Manual", "Message Queue"=w373) -> ()  [unwired: 7 in, 2 out]
          }
        }
      }
      frame "Reset Manual Count" {
        w378 = u32 0 ("Rejects")
        n157 = local write "Rejects 2"(w378) -> ()
        n158 = local write "Output Count"(w378) -> ()
      }
      frame "Reset AutoPause" {
        n159 = Variant To Data(error in=w391, type="" ("Message"), Variant=w389) -> (data=w387:string, error out=w390:errorcluster)
        n160 = case shown="\"ResetRejectCount\", Default" w387 {
          tunnel: w386 -> [w398 w403]
          tunnel: [w397 w402] -> w384
          tunnel: w385 -> [w396 w401]
          frame "ResetGoodCount" {
            n161 = Unbundle By Name(w396) -> ("General Para 2.OutputPause"=w395:dbl)
            n162 = To Unsigned Long Integer(number=w395) -> (unsigned 32bit integer=w394:u32)
            n163 = Bundle By Name(cluster=w398, "GoodPause"=w394) -> (w397:cluster{"GoodPause":u32, "RejectPause":u32})
          }
          frame "ResetRejectCount", Default {
            n164 = Unbundle By Name(w401) -> ("General Para 2.RejectPause"=w400:dbl)
            n165 = To Unsigned Long Integer(number=w400) -> (unsigned 32bit integer=w399:u32)
            n166 = Bundle By Name(cluster=w403, "RejectPause"=w399) -> (w402:cluster{"GoodPause":u32, "RejectPause":u32})
          }
        }
        n167 = Unbundle(w384) -> ("GoodPause"=w383:u32, "RejectPause"=w382:u32)
        n168 = local write "GoodPause"(w383) -> ()
        n169 = local write "RejectPause"(w382) -> ()
      }
      frame "Error" {
        w409 = 128  # call and forget
        # "Run async so that this loop will continue to run"
        # "Error"
        n170 = Variant To Data(error in=w428, type=errorcluster {"status"=FALSE, "code"=0, "source"=""} ("error constant"), Variant=w426) -> (data=w421:errorcluster, error out=w424:errorcluster)
        n171 = Unbundle By Name(w421) -> ("source"=w420:string)
        n172 = vi-ref "NewDialog.vi"() -> (w416:refnum<vi>)
        n173 = property class="VI"(reference=w416) -> (error out=w418:errorcluster, "Name"=w417:string)  [unwired: 1 in, 1 out]
        n174 = Search and Replace String(input string=w420, search string="<err>") -> (result string=w408:string)  [unwired: 6 in, 3 out]
        n175 = Open VI Reference(type specifier VI Refnum (for type only)=refnum<vi> refnum, vi path=w417, options=w409, error in (no error)=w418) -> (vi reference=w411:refnum<vi>, error out=w412:errorcluster)  [unwired: 2 in]
        n176 = call-by-ref "Start Asynchronous Call"(reference=w411, error in=w412, "inIcon"=T27."Error", "inTitle"="ERROR", "inMessage"=w408) -> (reference out=w414:refnum<vi>, error out=w413:errorcluster)  [unwired: 6 in, 3 out]
        n177 = Close Reference(reference=w414, error in (no error)=w413) -> (error out=w415:errorcluster)
        n178 = call <vilib>:"Simple Error Handler.vi"("error in (no error)"=w415) -> ()  [unwired: 4 in, 5 out]
        n179 = Merge Errors(w424) -> (w423:errorcluster)
      }
      frame "Confirm Quit" {
        # "Confirm Quit - Message that can confirm whether or not the user wants to exit the application."
        n180 = call "NewDialog.vi"("inIcon"=T27."Information", "inTitle"="SHUTDOWN?", "inButton2Text"="Shutdown", "inButton1Text"="", "inMessage"="Are you sure you want to shutdown?") -> ("outButton2"=w431:bool)  [unwired: 4 in, 2 out]
        "Shutdown?" <- w431
        n181 = case shown="True" w431 {
          tunnel: w442 -> [w443 w448]
          tunnel: [w443 w447] -> w439
          tunnel: w438 -> [_ w446]
          frame False {
          }
          frame True {
            n182 = call-poly "Enqueue Message.vi"("Priority Message? (F)"=TRUE, "error in (no error)"=w448, "Message"="Exit", "Message Queue"=w446) -> ("error out"=w447:errorcluster)  [unwired: 6 in, 1 out]
          }
        }
        n183 = Merge Errors(w439) -> (w440:errorcluster)
      }
      frame "Exit" {
        # "Stop the VI"
        # "Release the message queue reference"
        # "Exit - Exit the application."
        n184 = Variant To Data(type=errorcluster {"status"=FALSE, "code"=0, "source"=""} ("error constant"), Variant=w456) -> (data=w457:errorcluster)  [unwired: 1 in, 1 out]
        n185 = call <vilib>:"Simple Error Handler.vi"("error in (no error)"=w457) -> ()  [unwired: 4 in, 5 out]
        n186 = Send Notification(notification=TRUE, notifier=w455) -> (error out=w453:errorcluster)  [unwired: 1 in, 1 out]
        n187 = call "Fire User Event - Stop.vi"("User Event - Stop"=w461) -> ("error out"=w460:errorcluster)  [unwired: 10 in]
        n188 = Release Queue(queue=w466, error in (no error)=w459) -> (error out=w463:errorcluster)  [unwired: 1 in, 2 out]
        n189 = Merge Errors(w453, w460, w463) -> (w462:errorcluster)
        n190 = call "Stats Unbundle v0.2.vi"("State"=Logging_FGV."Save Values") -> ()  [unwired: 4 in, 7 out]
      }
      frame Default {
        # "'Default' case only runs if there is a message that isn't defined in any of the other cases.  Output a programming error."
        n191 = xnode "Error Ring"("parameter 0"=w470) -> ("error out"=w471:errorcluster)
      }
    }
    n192 = call "Error Handler - Message Handling Loop.vi"("error in (no error)"=w56, "Message Queue"=w58) -> ("dup error in"=w57:errorcluster)  [unwired: 8 in, 1 out]
  }
  n193 = while {
    tunnel: w33 -> [w488]
    shift-right: [w486] -> w39
    shift-left: w36 -> [w487]
    tunnel: [w482] -> w37
    tunnel: w3 -> [w480]
    stop <- w484 stop-if-true
    # "Event Handling Loop"
    n194 = event shown="[8] \"Home AC\": Value Change" {
      selector: w487 -> [_ _ _ _ _ _ _ _ _ _ _ _ _ _ _ _ _ _ _ _ _]
      dyn-events: [_ _ _ _ _ _ _ _ _ _ _ _ _ _ _ _ _ _ _ _ _] -> w486
      timeout: 500 -> [_ _ _ _ _ _ _ _ _ _ _ _ _ _ _ _ _ _ _ _ _]
      tunnel: [_ _ _ _ _ _ _ _ _ _ _ _ _ _ _ _ _ _ _ _ TRUE ("Discard?")] -> w484
      tunnel: w488 -> [w493 w497 w509 w514 w518 w522 w526 w530 w536 w541 w550 w574 w578 w582 w587 w589 w592 w623 w632 w641 w643]
      tunnel: [w492 _ _ w513 w517 w521 w525 w529 w535 w540 w549 w575 _ _ w585 w590 w595 _ _ _ _] -> w485
      tunnel: [w491 w497 w509 w512 w516 w520 w524 w528 w534 w539 w548 w574 w578 w582 w586 w589 w591 w623 w632 w641 w643] -> w483
      tunnel: w480 -> [_ _ _ _ _ _ _ _ _ _ w542 _ _ _ _ _ _ _ _ _ _]
      event Panel Close? {
        n195 = event-data() -> ()  [unwired: 1 in, 1 out]
        n196 = call-poly "Enqueue Message.vi"("Priority Message? (F)"=TRUE, "Message"="Exit", "Message Queue"=w493) -> ("error out"=w492:errorcluster, "dup Message Queue"=w491:refnum<queue>)  [unwired: 7 in]
        n197 = event-data("Discard?"=TRUE) -> ()  [unwired: 1 in, 1 out]
      }
      event Timeout {
        n198 = event-data() -> ()  [unwired: 1 in, 1 out]
        n199 = Format Date/Time String(time format string (%c)="%d %b %Y | %I:%M:%S %p") -> (date/time string=→"Date-Time":string)  [unwired: 2 in]
      }
      event "View Log": Value Change {
        w508 = 128  # call and forget
        n200 = event-data() -> ()  [unwired: 1 in, 1 out]
        n201 = local read "path"() -> (w498:path)
        n202 = vi-ref "View Log.vi"() -> (w501:refnum<vi>)
        n203 = property class="VI"(reference=w501) -> (error out=w499:errorcluster, "Name"=w500:string)  [unwired: 1 in, 1 out]
        n204 = Open VI Reference(type specifier VI Refnum (for type only)=refnum<vi> refnum, vi path=w500, options=w508, error in (no error)=w499) -> (vi reference=w506:refnum<vi>, error out=w505:errorcluster)  [unwired: 2 in]
        n205 = call-by-ref "Start Asynchronous Call"(reference=w506, error in=w505, "file path"=w498) -> (reference out=w503:refnum<vi>, error out=w504:errorcluster)  [unwired: 10 in, 1 out]
        n206 = Close Reference(reference=w503, error in (no error)=w504) -> (error out=w502:errorcluster)
        n207 = call <vilib>:"Simple Error Handler.vi"("error in (no error)"=w502) -> ()  [unwired: 4 in, 5 out]
      }
      event "Shutdown": Value Change {
        n208 = event-data() -> ()  [unwired: 1 in, 1 out]
        n209 = call-poly "Enqueue Message.vi"("Priority Message? (F)"=TRUE, "Message"="Confirm Quit", "Message Queue"=w514) -> ("error out"=w513:errorcluster, "dup Message Queue"=w512:refnum<queue>)  [unwired: 7 in]
      }
      event "Home Para", "Home Manual", "Home IOs": Value Change {
        n210 = event-data() -> ()  [unwired: 1 in, 1 out]
        n211 = call-poly "Enqueue Message.vi"("Message"="Initialize", "Message Queue"=w518) -> ("error out"=w517:errorcluster, "dup Message Queue"=w516:refnum<queue>)  [unwired: 8 in]
      }
      event "Back Stats", "Back IO": Value Change {
        n212 = event-data() -> ()  [unwired: 1 in, 1 out]
        n213 = call-poly "Enqueue Message.vi"("Message"="Autocycle Back", "Message Queue"=w522) -> ("error out"=w521:errorcluster, "dup Message Queue"=w520:refnum<queue>)  [unwired: 8 in]
      }
      event "Stats": Value Change {
        n214 = event-data() -> ()  [unwired: 1 in, 1 out]
        n215 = call-poly "Enqueue Message.vi"("Message"="Autocycle Stats", "Message Queue"=w526) -> ("error out"=w525:errorcluster, "dup Message Queue"=w524:refnum<queue>)  [unwired: 8 in]
      }
      event "All IO", "All IOs": Value Change {
        n216 = event-data() -> ()  [unwired: 1 in, 1 out]
        n217 = call-poly "Enqueue Message.vi"("Message"="Autocycle IO", "Message Queue"=w530) -> ("error out"=w529:errorcluster, "dup Message Queue"=w528:refnum<queue>)  [unwired: 8 in]
      }
      event "Home AC": Value Change {
        n218 = event-data() -> ()  [unwired: 1 in, 1 out]
        n219 = call-poly "Enqueue Message.vi"("Message"="Initialize", "Message Queue"=w536) -> ("error out"=w535:errorcluster, "dup Message Queue"=w534:refnum<queue>)  [unwired: 8 in]
        n220 = call "AVL Auto Time v0.1.vi"("State"=AVL_Auto_Time."Exited Auto") -> ()  [unwired: 9 in, 2 out]
        n221 = call "Write NS (HMI).vi"("Message"="Exit Autocycle") -> ()  [unwired: 10 in, 1 out]
      }
      event "Maintenance", "Manual": Value Change {
        n222 = event-data() -> ("CtlRef"=w538:refnum<vi>)  [unwired: 1 in]
        n223 = property class="Bool"(reference=w538) -> ("Label.Text"=w537:string)  [unwired: 1 in, 2 out]
        n224 = call-poly "Enqueue Message.vi"("Message"=w537, "Message Queue"=w541) -> ("error out"=w540:errorcluster, "dup Message Queue"=w539:refnum<queue>)  [unwired: 8 in]
      }
      event "Parameters": Value Change {
        n225 = event-data() -> ("CtlRef"=w547:refnum<vi>)  [unwired: 1 in, 2 out]
        n226 = call "HMI Pop Up Num KP v1.1.vi"("Password Display (F)"=FALSE, "Message In"="Please enter the passcode below:") -> ("Canceled"=w544:bool, "String Out"=w543:string)  [unwired: 8 in]
        n227 = case shown="False" w544 {
          tunnel: w550 -> [w557 w569]
          tunnel: [w556 _] -> w549
          tunnel: [w555 w569] -> w548
          tunnel: w547 -> [w554 _]
          tunnel: w543 -> [w553 _]
          tunnel: w542 -> [w552 _]
          frame False {
            n228 = Equal?(x=w553, y=w552) -> (x = y?=w551:bool)
            n229 = case shown="False" w551 {
              tunnel: w557 -> [w562 w567]
              tunnel: [w561 w566] -> w556
              tunnel: [w560 w565] -> w555
              tunnel: w554 -> [w559 _]
              frame True {
                n230 = property class="Bool"(reference=w559) -> ("Label.Text"=w558:string)  [unwired: 1 in, 2 out]
                n231 = call-poly "Enqueue Message.vi"("Message"=w558, "Message Queue"=w562) -> ("error out"=w561:errorcluster, "dup Message Queue"=w560:refnum<queue>)  [unwired: 8 in]
              }
              frame False {
                n232 = xnode "Error Ring"() -> ("error out"=w563:errorcluster)
                n233 = call-poly "Enqueue Message.vi"("Message Data"=w563, "Message"="Error" ("Message In"), "Message Queue"=w567) -> ("error out"=w566:errorcluster, "dup Message Queue"=w565:refnum<queue>)  [unwired: 7 in]
              }
            }
          }
          frame True {
          }
        }
      }
      event "End Cycle", "Enable Cutting?", "Enable TF?", "Enable PF?", "Enable Index?", "Enable Measure?", "Enable Reject?", "Enable Agitate?", "Enable BF?", "Enable Insertion?": Value Change {
        n234 = event-data() -> ("CtlRef"=w576:refnum<vi>, "NewVal"=w570:bool)  [unwired: 1 in, 1 out]
        n235 = property class="Bool"(reference=w576) -> ("Label.Text"=w573:string)  [unwired: 1 in, 2 out]
        n236 = Concatenate Strings("GV:" ("string"), w573) -> (w571:string)
        n237 = call "Write NS (HMI).vi"("Message Data"=w570, "Message"=w571) -> ("error out"=w575:errorcluster)  [unwired: 9 in]
      }
      event "Reset MCount": Value Change {
        n238 = event-data() -> ()  [unwired: 1 in, 6 out]
        n239 = call-poly "Enqueue Message.vi"("Message"="Reset Manual Count", "Message Queue"=w578) -> ()  [unwired: 8 in, 2 out]
      }
      event "ResetGoodCount", "ResetRejectCount": Value Change {
        n240 = event-data() -> ("CtlRef"=w580:refnum<vi>)  [unwired: 1 in]
        n241 = property class="Bool"(reference=w580) -> ("Label.Text"=w579:string)  [unwired: 1 in, 2 out]
        n242 = call-poly "Enqueue Message.vi"("Message Data"=w579, "Message"="Reset AutoPause", "Message Queue"=w582) -> ()  [unwired: 7 in, 2 out]
      }
      event "Run Manual": Value Change {
        n243 = event-data() -> ("CtlRef"=w584:refnum<vi>)  [unwired: 1 in, 2 out]
        n244 = property class="Bool"(reference=w584) -> ("Label.Text"=w583:string)  [unwired: 1 in, 2 out]
        n245 = call-poly "Enqueue Message.vi"("Message"=w583, "Message Queue"=w587) -> ("error out"=w585:errorcluster, "dup Message Queue"=w586:refnum<queue>)  [unwired: 8 in]
      }
      event "Toggle Motor": Value Change {
        n246 = event-data() -> ()  [unwired: 1 in, 3 out]
        n247 = call "Write NS (HMI).vi"("Message"="Toggle Motor") -> ("error out"=w590:errorcluster)  [unwired: 10 in]
      }
      event "Save Para": Value Change {
        n248 = event-data() -> ()  [unwired: 1 in, 3 out]
        n249 = Cluster To Array(cluster="Agitator Para") -> (array=w612:u32[])
        n250 = Cluster To Array(cluster="Tube Feeder Para") -> (array=w610:u32[])
        n251 = Cluster To Array(cluster="Insertion Para") -> (array=w608:u32[])
        n252 = Cluster To Array(cluster="Cutting Para") -> (array=w606:u32[])
        n253 = Cluster To Array(cluster="PF Para") -> (array=w604:u32[])
        n254 = Cluster To Array(cluster="Meas. Para") -> (array=w602:dbl[])
        n255 = Cluster To Array(cluster="Reject Para") -> (array=w600:u32[])
        n256 = Cluster To Array(cluster="BF Para") -> (array=w598:u32[])
        n257 = Bundle By Name(cluster=T8 {"Agitator Delays"=[1000], "TF Delays"=[1000], "Insertion Delays"=[1000], "Cutting Delays"=[1000], "PF Delays"=[1000], "Measur. Delays"=[1000.0], "Reject Delays"=[1000], "BF Delays"=[1000]} ("Auto Para"), "Agitator Delays"=w612, "TF Delays"=w610, "Insertion Delays"=w608, "Cutting Delays"=w606, "PF Delays"=w604, "Measur. Delays"=w602, "Reject Delays"=w600, "BF Delays"=w598) -> (w597:T8)
        n258 = Bundle("Auto Para"=w597, "General Para"="General Para") -> (w594:cluster{"Auto Para":T8, "General Para":T4})  [unwired: 1 in]
        n259 = property on="Auto Para" class="Clust (strict)"("Value"=w597) -> ()  [unwired: 2 in, 2 out]
        n260 = call-poly "Enqueue Message.vi"("Message Data"=w594, "Message"="Update Para", "Message Queue"=w592) -> ("error out"=w595:errorcluster, "dup Message Queue"=w591:refnum<queue>)  [unwired: 7 in]
      }
      event "Insertion Para.Delay 1", "Insertion Para.Delay 2", "Agitator Para.Delay 1", "Agitator Para.Delay 2", "Cutting Para.Delay", "Cutting Para.Delay 2", "Cutting Para.Delay 3", "Tube Feeder Para.Delay", "Tube Feeder Para.Delay 2", "Tube Feeder Para.Max Attempts", "PF Para.Delay 1", "PF Para.Delay 2", "Reject Para.Delay", "BF Para.Delay 1", "BF Para.Delay 2", "Tube Feeder Para.Timeout": Mouse Up {
        n261 = event-data() -> ("CtlRef"=w615:refnum<vi>)  [unwired: 1 in, 4 out]
        n262 = property class="DigNum (strict)"(reference=w615) -> (reference out=w618:refnum<vi>, "Value"=w619:u32)  [unwired: 1 in, 1 out]
        n263 = Number To Fractional String(number=w619, precision (6)=0.0 ("width (-)")) -> (F-format string=w617:string)  [unwired: 2 in]
        n264 = call "HMI Pop Up Num KP v1.1.vi"("String In"=w617) -> ("String Out"=w616:string)  [unwired: 9 in, 1 out]
        n265 = Fract/Exp String To Number(string=w616, default (0 dbl)=0.0 ("default (0 I32)")) -> (number=w621:dbl)  [unwired: 2 in, 1 out]
        n266 = property class="DigNum (strict)"(reference=w618, "Value"=w621) -> ()  [unwired: 1 in, 2 out]
      }
      event "Meas. Para.Delay": Mouse Up {
        n267 = event-data() -> ("CtlRef"=w624:refnum<vi>)  [unwired: 1 in, 4 out]
        n268 = property class="DigNum (strict)"(reference=w624) -> (reference out=w627:refnum<vi>, "Value"=w628:dbl)  [unwired: 1 in, 1 out]
        n269 = Number To Fractional String(number=w628, precision (6)=0.0 ("width (-)")) -> (F-format string=w626:string)  [unwired: 2 in]
        n270 = call "HMI Pop Up Num KP v1.1.vi"("String In"=w626) -> ("String Out"=w625:string)  [unwired: 9 in, 1 out]
        n271 = Fract/Exp String To Number(string=w625, default (0 dbl)=0.0 ("default (0 I32)")) -> (number=w630:dbl)  [unwired: 2 in, 1 out]
        n272 = property class="DigNum (strict)"(reference=w627, "Value"=w630) -> ()  [unwired: 1 in, 2 out]
      }
      event "Meas. Para.Mean Length", "Meas. Para.Tolerance": Mouse Up {
        n273 = event-data() -> ("CtlRef"=w633:refnum<vi>)  [unwired: 1 in, 4 out]
        n274 = property class="DigNum (strict)"(reference=w633) -> (reference out=w636:refnum<vi>, "Value"=w637:dbl)  [unwired: 1 in, 1 out]
        n275 = Number To Fractional String(number=w637, precision (6)=2.0 ("width (-)")) -> (F-format string=w635:string)  [unwired: 2 in]
        n276 = call "HMI Pop Up Num KP v1.1.vi"("String In"=w635) -> ("String Out"=w634:string)  [unwired: 9 in, 1 out]
        n277 = Fract/Exp String To Number(string=w634, default (0 dbl)=0.0 ("default (0 I32)")) -> (number=w639:dbl)  [unwired: 2 in, 1 out]
        n278 = property class="DigNum (strict)"(reference=w636, "Value"=w639) -> ()  [unwired: 1 in, 2 out]
      }
      event User Event {
        # "The Message Handling Loop processed an \"Exit\" message, which fired this event to stop the Event Handling Loop."
        n279 = event-data() -> ()  [unwired: 1 in, 1 out]
      }
    }
    n280 = call "Error Handler - Event Handling Loop.vi"("error in (no error)"=w485, "Message Queue"=w483) -> ("dup error in"=w482:errorcluster)  [unwired: 8 in, 1 out]
  }
  n281 = call "HMI-cRIO Connection Manager.vi"("error in"=w2, "notifier in"=w7, "Queue in"=w33) -> ("error out"=w27:errorcluster, "Notifier out"=w28:refnum<notifier>)  [unwired: 7 in]
  n282 = Unregister For Events(event registration refnum=w39, error in=w37) -> (error out=w40:errorcluster)
  n283 = Merge Errors(w40, w42, w27) -> (w41:errorcluster)
  n284 = call "Destroy User Event - Stop.vi"("error in (no error)"=w41, "User Event - Stop"=w35) -> ("error out"=w30:errorcluster)  [unwired: 9 in]
  n285 = Release Notifier(notifier=w28, error in (no error)=w30) -> (error out=w29:errorcluster)  [unwired: 1 in, 2 out]
  n286 = disable-structure shown="RUN_TIME_ENGINE==True" {
    disable-tunnel: w29 -> [_ _]
    frame condition #0 (active) {
    }
    frame condition #1 {
      n287 = local read "Shutdown?"() -> (w644:bool)
      n288 = case shown="True" w644 {
        tunnel: [_ w646] -> w645
        frame False {
        }
        frame True {
          n289 = call <vilib>:"System Exec.vi"("wait until completion? (T)"=TRUE, "command line"="Shutdown -s -f -t 10") -> ("error out"=w646:errorcluster)  [unwired: 6 in, 3 out]
        }
      }
      n290 = flat-sequence {
        tunnel: w645 -> [_]
        frame #0 {
          n291 = Quit LabVIEW() -> ()  [unwired: 1 in]
        }
      }
    }
  }
